vi "CreateProduct.vi"(8 "error in (no error)":errorcluster, 11 "ProductA_Factory in":refnum<class "ProductA_Factory.lvclass">) -> (0 "error out":errorcluster, 2 "Product.lvclass":refnum<class "Product.lvclass">, 3 "ProductA_Factory out":refnum<class "ProductA_Factory.lvclass">)   [LabVIEW 2016, in "ProductA_Factory.lvclass"]
uses:
  Product Class/ProductA_Factory.lvclass
  Product Class/Product/Product.lvclass
  Product Class/ProductA/ProductA.lvclass
  C:/Users/Felipe/Desktop/LabVIEW OOP Design Patters Folder/LabVIEW OOP Design Patters Folder/Factory Method Pattern/Product Class/Product/Product.lvclass
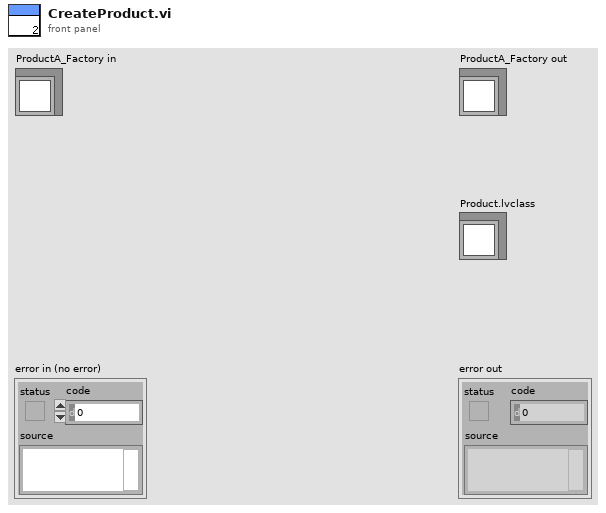
[diagram p1: front panel]
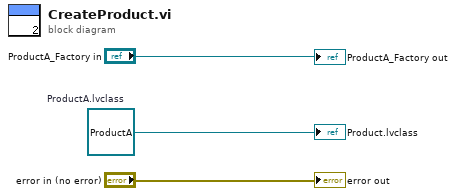
[diagram p0: block diagram]
diagram:
  w1 = refnum<class "ProductA.lvclass"> refnum  # ProductA.lvclass
  "error out" <- "error in (no error)"
  "ProductA_Factory out" <- "ProductA_Factory in"
  "Product.lvclass" <- w1
